vi "Data Log.vi"   [LabVIEW 2021]
doc: "This VI manages the data logging operation."
uses:
  Controls/DataLog.ctl
  support/Message Queue/Enqueue Message (Single).vi
  <vilib>/Utility/file.llb/Write Delimited Spreadsheet (string).vi
  <vilib>/Utility/file.llb/Read Delimited Spreadsheet (string).vi
  <vilib>/Utility/error.llb/Error Cluster From Error Code.vi
  <vilib>/ErrorRing/Error Ring.xnode
  support/Message Queue/Message Queue.lvlib
  support/User Event - Stop/User Event - Stop.lvlib
types:
  T1 = typedef "DataLog.ctl" = cluster{"Status":string, "Log File Path":path}
  T2 = enum32{"No Selection", "Serial", "TCP", "Modbus"}
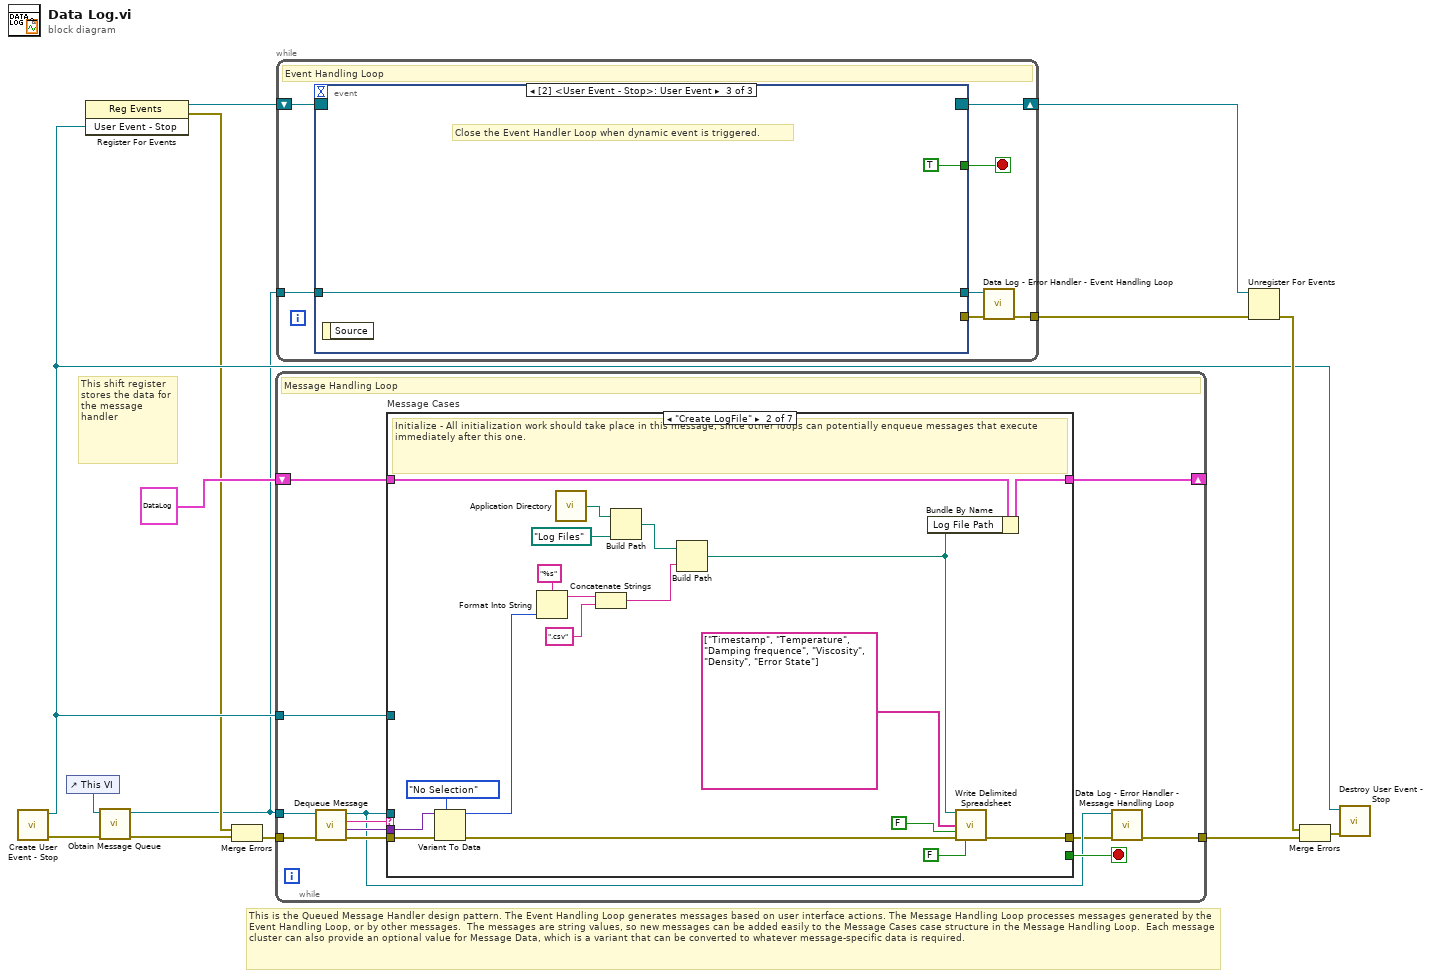
[diagram p0: block diagram]
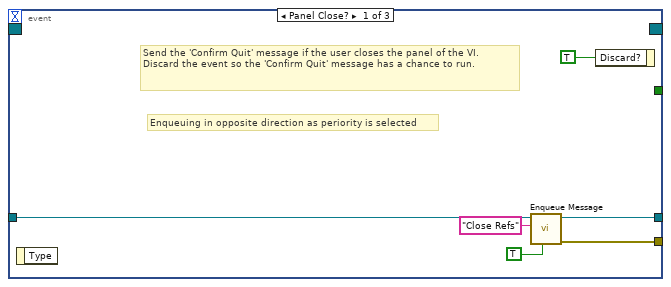
[diagram p2: hidden frame]
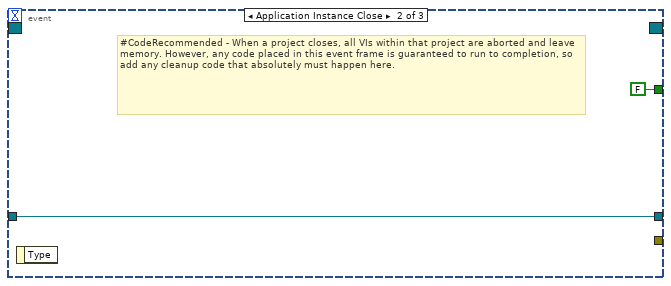
[diagram p3: hidden frame]
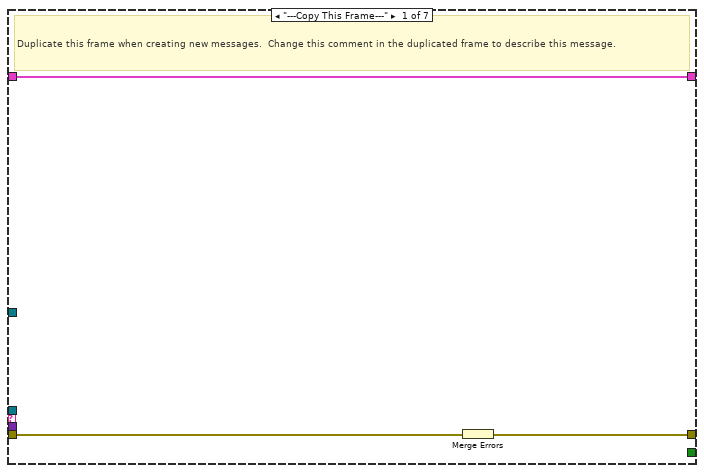
[diagram p4: hidden frame]
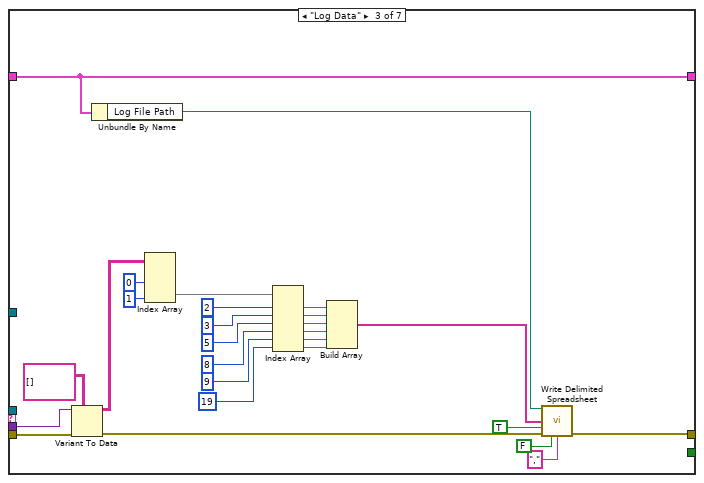
[diagram p5: hidden frame]
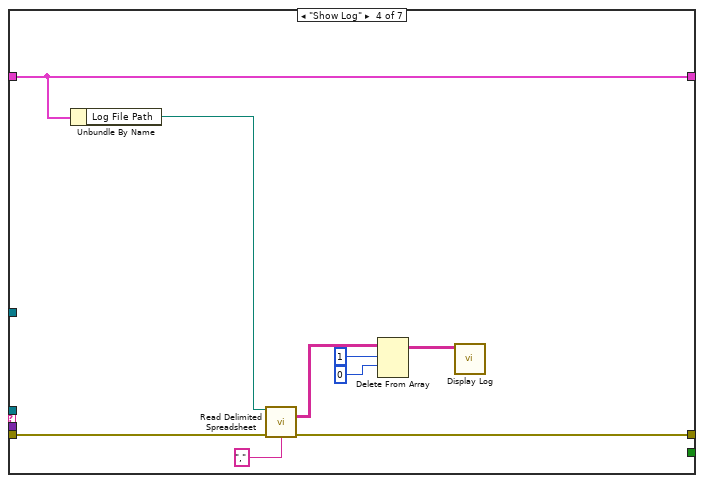
[diagram p6: hidden frame]
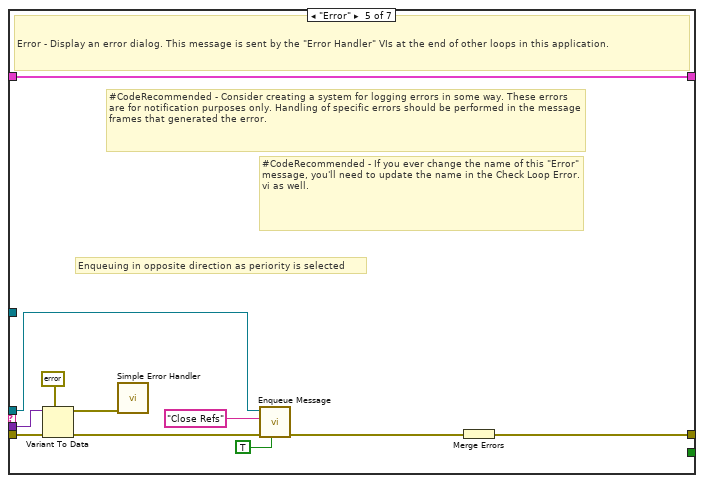
[diagram p7: hidden frame]
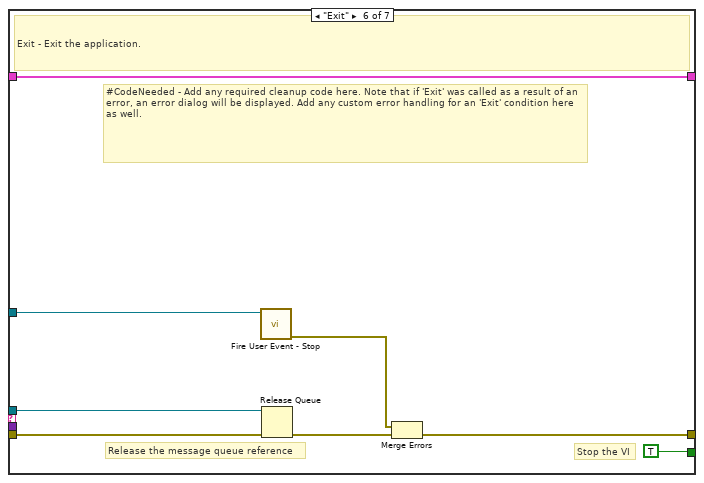
[diagram p8: hidden frame]
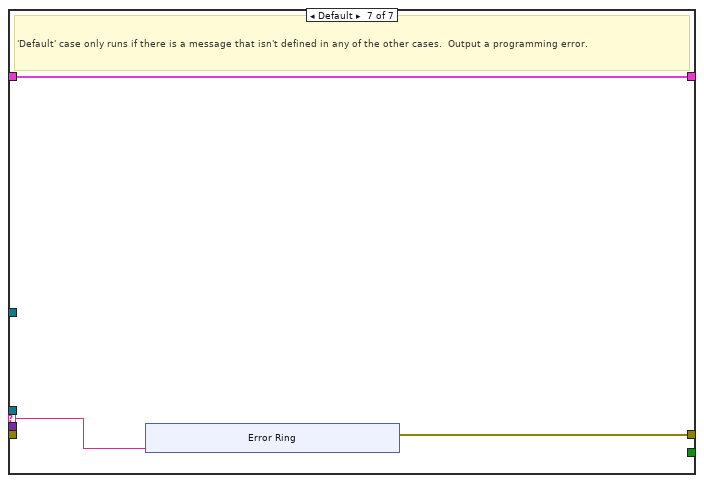
[diagram p9: hidden frame]
diagram:
  # "This is the Queued Message Handler design pattern. The Event Handling Loop generates messages based on user interface actions. The Message Handling Loop processes messages generated by the Event Handling Loop, or by other messages.  The messages are string values, so new messages can be added easily to the Message Cases case structure in the Message Handling Loop.  Each message cluster can also provide an optional value for Message Data, which is a variant that can be converted to whatever message-specific data is required."
  # "This shift register stores the data for the message handler"
  n1 = call "Create User Event - Stop.vi"() -> ("error out"=w4:errorcluster, "User Event - Stop"=w7:refnum<user-event>)  [unwired: 10 in]
  n2 = control-ref of="This VI"() -> (w3:refnum<vi>)
  n3 = register-events(w7) -> (reference out=w8:refnum<event-registration>, error out=w5:errorcluster)  [unwired: 2 in]
  n4 = call "Obtain Message Queue.vi"("error in"=w4, "VI Ref"=w3) -> ("error out"=w1:errorcluster, "Message Queue"=w2:refnum<queue>)  [unwired: 8 in]
  n5 = Merge Errors(w5, w1) -> (w6:errorcluster)
  n6 = while {
    tunnel: w2 -> [w18]
    shift-right: [w25] -> _
    shift-left: T1 {"Status"="", "Log File Path"=path "Data Log/Log Files/Log.csv"} ("Data Cluster") -> [w26]
    tunnel: w7 -> [w23]
    tunnel: w6 -> [w22]
    tunnel: [w15] -> w14
    stop <- w24 stop-if-true
    # "Message Handling Loop"
    n7 = call "Dequeue Message.vi"("error in (no error)"=w22, "Message Queue"=w18) -> ("error out"=w21:errorcluster, "Message Data"=w19:variant, "Message"=w20:string, "dup Message Queue"=w17:refnum<queue>)  [unwired: 6 in]
    n8 = case "Message Cases" shown="\"Create LogFile\"" w20 {
      selector: w20 -> [_ _ _ _ _ _ w104]
      tunnel: w17 -> [_ _ _ _ w87 w103 _]
      tunnel: w21 -> [w29 w41 w74 w83 w95 w96 _]
      tunnel: [w27 w47 w75 w82 w90 w99 w105] -> w16
      tunnel: w26 -> [w28 w48 w65 w84 w94 w102 w106]
      tunnel: [w28 w44 w65 w84 w94 w102 w106] -> w25
      tunnel: [_ _ _ _ _ TRUE _] -> w24
      tunnel: w19 -> [_ w38 w72 _ w93 _ _]
      tunnel: w23 -> [_ _ _ _ _ w98 _]
      frame "---Copy This Frame---" {
        # "Duplicate this frame when creating new messages.  Change this comment in the duplicated frame to describe this message."
        n9 = Merge Errors(w29) -> (w27:errorcluster)
      }
      frame "Create LogFile" {
        # "Initialize - All initialization work should take place in this message, since other loops can potentially enqueue messages that execute immediately after this one."
        n10 = Variant To Data(error in=w41, type=T2."No Selection" ("ProtocolSelect"), Variant=w38) -> (data=w35:T2, error out=w40:errorcluster)
        n11 = Format Into String(format string="%s", w35) -> (resulting string=w33:string)  [unwired: 2 in, 1 out]
        n12 = call <vilib>:"Application Directory.vi"() -> ("Application Directory"=w46:path)
        n13 = Concatenate Strings(w33, ".csv" ("string")) -> (w32:string)
        n14 = Build Path(base path=w46, name or relative path=path "Log Files") -> (appended path=w37:path)
        n15 = Build Path(base path=w37, name or relative path=w32) -> (appended path=w36:path)
        n16 = Bundle By Name(cluster=w48, "Log File Path"=w36) -> (w44:T1)
        n17 = call-poly <vilib>:"Write Delimited Spreadsheet.vi"("file path (dialog if empty)"=w36, "1D data"=string[] ["Timestamp", "Temperature", "Damping frequence", "Viscosity", "Density", "Error State"], "append to file? (new file:F)"=FALSE, "error in (no error)"=w40, "transpose? (no:F)"=FALSE) -> ("error out"=w47:errorcluster)  [unwired: 9 in, 1 out]
      }
      frame "Log Data" {
        n18 = Variant To Data(error in=w74, type=string[][] [], Variant=w72) -> (data=w68:string[][], error out=w73:errorcluster)
        n19 = Unbundle By Name(w65) -> ("Log File Path"=w64:path)
        n20 = Index Array(array=w68, index (col) #1=0 ("disabled index (col)"), index (col) #2=1 ("index (col)")) -> (element #2=w63:string[])  [unwired: 2 in, 1 out]
        n21 = Index Array(array=w63, index #1=2 ("index"), index #2=3 ("index"), index #3=5 ("index"), index #4=8 ("index"), index #5=9 ("index"), index #6=19 ("index")) -> (element #1=w56:string, element #2=w55:string, element #3=w54:string, element #4=w53:string, element #5=w52:string, element #6=w51:string)
        n22 = Build Array(w56, w55, w54, w53, w52, w51) -> (w49:string[])
        n23 = call-poly <vilib>:"Write Delimited Spreadsheet.vi"("file path (dialog if empty)"=w64, "1D data"=w49, "append to file? (new file:F)"=TRUE, "error in (no error)"=w73, "transpose? (no:F)"=FALSE, "delimiter (\\t)"="," ("delimiter (\\t)")) -> ("error out"=w75:errorcluster)  [unwired: 8 in, 1 out]
      }
      frame "Show Log" {
        n24 = Unbundle By Name(w84) -> ("Log File Path"=w80:path)
        n25 = call-poly <vilib>:"Read Delimited Spreadsheet.vi"("file path (dialog if empty)"=w80, "error in (no error)"=w83, "delimiter (\\t)"="," ("delimiter (\\t)")) -> ("all rows"=w79:string[][], "error out"=w82:errorcluster)  [unwired: 7 in, 4 out]
        n26 = Delete From Array(array=w79, length=1, index (row)=0) -> (array with subset deleted=w78:string[][])  [unwired: 1 in, 1 out]
        n27 = call "Display Log.vi"("all rows"=w78) -> ()  [unwired: 11 in]
      }
      frame "Error" {
        # "Enqueuing in opposite direction as periority is selected"
        # "#CodeRecommended - If you ever change the name of this \"Error\" message, you'll need to update the name in the Check Loop Error.vi as well."
        # "#CodeRecommended - Consider creating a system for logging errors in some way. These errors are for notification purposes only. Handling of specific errors should be performed in the message frames that generated the error."
        # "Error - Display an error dialog. This message is sent by the \"Error Handler\" VIs at the end of other loops in this application."
        n28 = Variant To Data(error in=w95, type=errorcluster {"status"=FALSE, "code"=0, "source"=""} ("error constant"), Variant=w93) -> (data=w91:errorcluster, error out=w89:errorcluster)
        n29 = call <vilib>:"Simple Error Handler.vi"("error in (no error)"=w91) -> ()  [unwired: 4 in, 5 out]
        n30 = call-poly "Enqueue Message.vi"("Priority Message? (F)"=TRUE, "error in (no error)"=w89, "Message"="Close Refs", "Message Queue"=w87) -> ("error out"=w88:errorcluster)  [unwired: 6 in, 1 out]
        n31 = Merge Errors(w88) -> (w90:errorcluster)
      }
      frame "Exit" {
        # "Stop the VI"
        # "Release the message queue reference"
        # "#CodeNeeded - Add any required cleanup code here. Note that if 'Exit' was called as a result of an error, an error dialog will be displayed. Add any custom error handling for an 'Exit' condition here as well."
        # "Exit - Exit the application."
        n32 = call "Fire User Event - Stop.vi"("User Event - Stop"=w98) -> ("error out"=w97:errorcluster)  [unwired: 10 in]
        n33 = Release Queue(queue=w103, error in (no error)=w96) -> (error out=w100:errorcluster)  [unwired: 1 in, 2 out]
        n34 = Merge Errors(w97, w100) -> (w99:errorcluster)
      }
      frame Default {
        # "'Default' case only runs if there is a message that isn't defined in any of the other cases.  Output a programming error."
        n35 = xnode "Error Ring"("parameter 0"=w104) -> ("error out"=w105:errorcluster)
      }
    }
    n36 = call "Data Log - Error Handler - Message Handling Loop.vi"("error in (no error)"=w16, "Message Queue"=w17) -> ("dup error in"=w15:errorcluster)  [unwired: 8 in, 1 out]
  }
  n37 = while {
    tunnel: w2 -> [w120]
    shift-right: [w118] -> w11
    shift-left: w8 -> [w119]
    tunnel: [w114] -> w9
    stop <- w117 stop-if-true
    # "Event Handling Loop"
    n38 = event shown="[2] <User Event - Stop>: User Event" {
      selector: w119 -> [_ _ _]
      dyn-events: [_ _ _] -> w118
      timeout: _ -> [_ _ _]
      tunnel: [_ FALSE ("Discard?") TRUE ("Discard?")] -> w117
      tunnel: w120 -> [w125 w128 w130]
      tunnel: [w124 _ _] -> w115
      tunnel: [w123 w128 w130] -> w116
      event Panel Close? {
        # "Enqueuing in opposite direction as periority is selected"
        # "Send the 'Confirm Quit' message if the user closes the panel of the VI. Discard the event so the 'Confirm Quit' message has a chance to run."
        n39 = event-data() -> ()  [unwired: 1 in, 1 out]
        n40 = call-poly "Enqueue Message.vi"("Priority Message? (F)"=TRUE, "Message"="Close Refs", "Message Queue"=w125) -> ("error out"=w124:errorcluster, "dup Message Queue"=w123:refnum<queue>)  [unwired: 7 in]
        n41 = event-data("Discard?"=TRUE) -> ()  [unwired: 1 in, 1 out]
      }
      event Application Instance Close {
        # "#CodeRecommended - When a project closes, all VIs within that project are aborted and leave memory. However, any code placed in this event frame is guaranteed to run to completion, so add any cleanup code that absolutely must happen here."
        n42 = event-data() -> ()  [unwired: 1 in, 1 out]
      }
      event User Event {
        # "Close the Event Handler Loop when dynamic event is triggered."
        n43 = event-data() -> ()  [unwired: 1 in, 1 out]
      }
    }
    n44 = call "Data Log - Error Handler - Event Handling Loop.vi"("error in (no error)"=w115, "Message Queue"=w116) -> ("dup error in"=w114:errorcluster)  [unwired: 8 in, 1 out]
  }
  n45 = Unregister For Events(event registration refnum=w11, error in=w9) -> (error out=w12:errorcluster)
  n46 = Merge Errors(w12, w14) -> (w13:errorcluster)
  n47 = call "Destroy User Event - Stop.vi"("error in (no error)"=w13, "User Event - Stop"=w7) -> ()  [unwired: 9 in, 1 out]
